vi "Do.vi"(8 "error in (no error)":errorcluster, 10 "Actor in":refnum<class "Actor.lvclass">, 11 "Analyze Msg":refnum<class "Analyze Msg.lvclass">) -> (0 "error out":errorcluster, 2 "Actor out":refnum<class "Actor.lvclass">)   [LabVIEW 2020, in "Analyze Actor.lvlib" / "Analyze Msg.lvclass"]
doc: "This VI delivers the message to the actor by calling the appropriate method(s) on the actor."
uses:
  Analyze Msg.lvclass
  <vilib>/ActorFramework/Actor/Actor.lvclass
  Analyze Actor/Analyze Actor.lvclass
  C:/Program Files (x86)/National Instruments/LabVIEW 2020/vi.lib/ActorFramework/Actor/Actor.lvclass
  Analyze Msg.lvclass/Analyze Msg.ctl
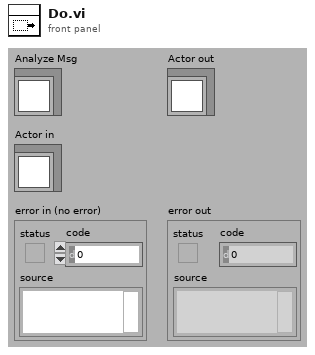
[diagram p1: front panel]
types:
  T1 = typedef "Analyze Actor.lvlib/Analyze Actor.lvclass/Analyze.ctl" = cluster{"Image":T2, "ImageNr":i32, "Analyze Objects":refnum<class "Analyze BaseClass.lvclass">[], "Pre Results":refnum<class "Analyze Results Base.lvclass">[]}
  T2 = typedef "IMAQ Image.ctl" = refnum<image>
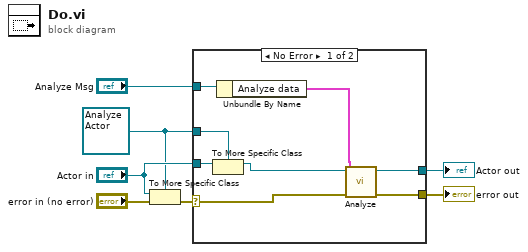
[diagram p0: block diagram]
diagram:
  w2 = refnum<class "Analyze Actor.lvclass"> refnum ("Actor in")
  n1 = To More Specific Class(target class=w2, reference="Actor in", error in="error in (no error)") -> (error out=w6:errorcluster)  [unwired: 1 out]
  n2 = case shown="No Error" w6 {
    selector: w6 -> [w12 w17]
    tunnel: [w11 w17] -> w5
    tunnel: [w10 w16] -> w4
    tunnel: "Actor in" -> [w15 w16]
    tunnel: w2 -> [w14 _]
    tunnel: "Analyze Msg" -> [w9 _]
    frame No Error {
      n3 = To More Specific Class(target class=w14, reference=w15) -> (specific class reference=w13:refnum<class "Analyze Actor.lvclass">)  [unwired: 1 in, 1 out]
      n4 = Unbundle By Name(w9) -> ("Analyze data"=w8:T1)
      n5 = call-dynamic "Analyze.vi"("error in (no error)"=w12, "Analyze Data"=w8, "Analyze Actor.lvlib:Analyze Actor.lvclass"=w13) -> ("error out"=w11:errorcluster, "Analyze Actor.lvlib:Analyze Acto out"=w10:refnum<class "Analyze Actor.lvclass">)  [unwired: 7 in]
    }
    frame Error {
      # "If type check fails, pass the original object out again."
    }
  }
  "error out" <- w5
  "Actor out" <- w4
